vi "open.vi"(8 "error in (no error)":errorcluster, 11 "reference":refnum<visa-resource-name>) -> (0 "error out":errorcluster, 3 "reference out":refnum<visa-resource-name>)   [LabVIEW 2017]
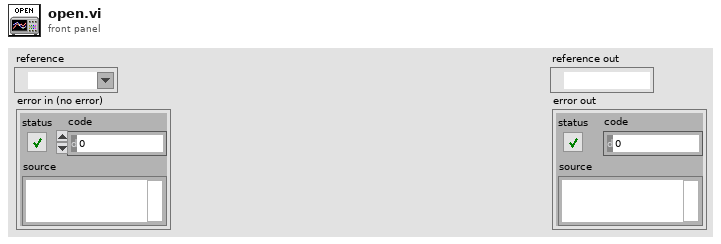
[diagram p1: front panel]
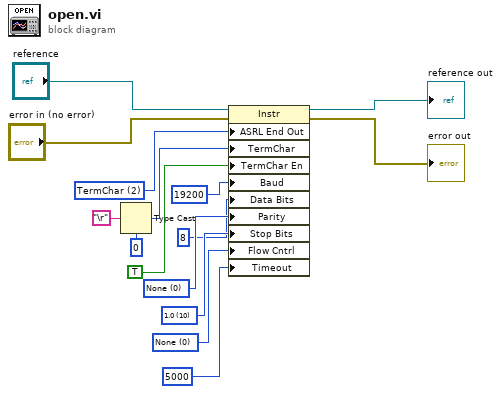
[diagram p0: block diagram]
diagram:
  w14 = u16 0 items=["None", "XON/XOFF", "RTS/CTS", "XON/XOFF & RTS/CTS", "DTR/DSR", "XON/XOFF & DTR/DSR"] ("Serial Settings:Flow Control")
  w13 = u16 10 items=["1.0"=10, "1.5"=15, "2.0"=20] ("Serial Settings:Stop Bits")
  w12 = u16 0 items=["None", "Odd", "Even", "Mark", "Space"] ("Serial Settings:Parity")
  w5 = u16 2 items=["None", "Last Bit", "TermChar", "Break"] ("Serial Settings:End Mode for Writes")
  n1 = Type Cast(type=u8 0 ("Message Based Settings:Termination Character"), x="\r") -> (*(type *) &x=w8:u8)
  n2 = property class="Instr"(reference="reference", error in="error in (no error)", "ASRL End Out"=w5, "TermChar"=w8, "TermChar En"=TRUE ("Message Based Settings:Termination Character Enable"), "Baud"=u32 19200 ("Serial Settings:Baud Rate"), "Data Bits"=u16 8 ("Serial Settings:Data Bits"), "Parity"=w12, "Stop Bits"=w13, "Flow Cntrl"=w14, "Timeout"=u32 5000 ("General Settings:Timeout Value")) -> (reference out=→"reference out":refnum<visa-resource-name>, error out=→"error out":errorcluster)
